vi "HGF_DIMSubscriber.appendData2Variant.vi"(0 "initData":variant, 2 "typeOfDimService (monitored)":T1=4 items=["ONCE_ONLY"=1, "TIMED"=2, "MONITORED"=4], 3 "timeout [0s]":i32, 4 "stamped (T)":bool=TRUE, 5 "error in (no error)":errorcluster) -> (14 "dup initData":variant, 19 "error out":errorcluster)   [LabVIEW 2012, in "HGF_DIM.lvlib" / "HGF_DIMSubscriber.lvclass"]
uses:
  HGF_DIMSubscriber.lvclass
  DimLVEvent/LVDimInterface/LVDimInterface.dim service type.ctl
  DimLVEvent/LVDimInterface/LVDimInterface.lvlib
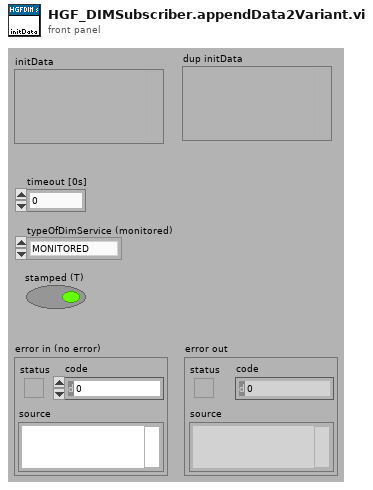
[diagram p1: front panel]
types:
  T1 = typedef "LVDimInterface.lvlib/LVDimInterface.dim service type.ctl" = u16
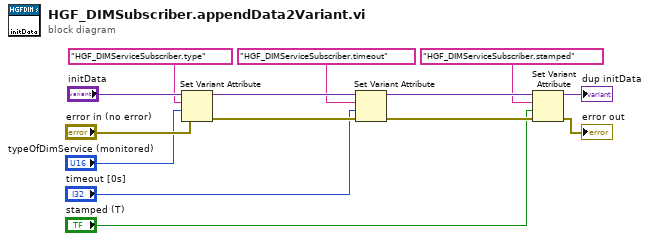
[diagram p0: block diagram]
diagram:
  n1 = Set Variant Attribute(Variant="initData", name="HGF_DIMServiceSubscriber.type", value="typeOfDimService (monitored)", error in="error in (no error)") -> (Variant out=w9:variant, error out=w7:errorcluster)  [unwired: 1 out]
  n2 = Set Variant Attribute(Variant=w9, name="HGF_DIMServiceSubscriber.timeout", value="timeout [0s]", error in=w7) -> (Variant out=w8:variant, error out=w6:errorcluster)  [unwired: 1 out]
  n3 = Set Variant Attribute(Variant=w8, name="HGF_DIMServiceSubscriber.stamped", value="stamped (T)", error in=w6) -> (Variant out=→"dup initData":variant, error out=→"error out":errorcluster)  [unwired: 1 out]
